vi "Graph of Function and Derivative.vi"() -> ()   [LabVIEW 2020, in "Examples.lvlib"]
doc: "A simple example demonstrating the easiness and usefulness of being able to calculate the derivative of a function automatically, even exchanging which function to differentiate at run-time. This example shows the graph of two different functions and plots the tangent line to the curve at the location of the cursor."
uses:
  Examples.lvlib
  classes/Dual/Dual.lvclass/Dual.ctl
  classes/Dual/Dual to Double.vi
  Automatic Differentiation/Evaluate Function.vi/9b1629ae-3de0-49eb-9b0a-cc9e581fb6c0.vi
  classes/Dual/Add infinitesimal to Double.vi
  classes/Dual/Read Dual Part.vi
  Automatic Differentiation/Evaluate Function.vi/9b1629ae-3de0-49eb-9b0a-cc9e581fb6c0.vi/5957e011-cf56-4527-b6ed-13c3a4ca997b.vi
  classes/Dual/Write a.vi
  Quadratic Function.vi
  Cubic Function.vi
  classes/Dual/Dual.lvclass
  Automatic Differentiation/Automatic Differentiation.lvlib
panel:
  in  "Toggle Function":bool
  in  "Stop":bool
  out "XY Graph":cluster{dbl[], dbl[]}[](graph)
  # "1) Run the VI\n2) Grab and move the cursor and view the graph of the tangent line changing\n3) Toggle f(x) to change the function at run-time\n4) Inspect the block diagram"
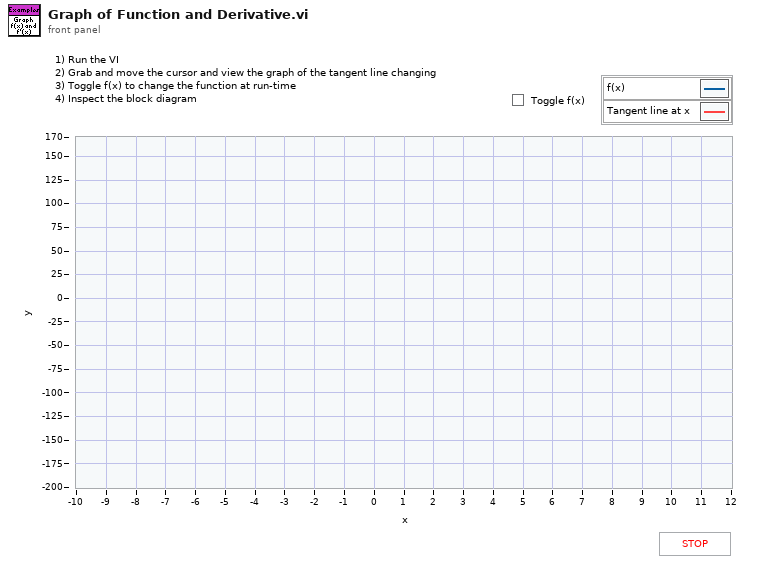
[diagram p1: front panel]
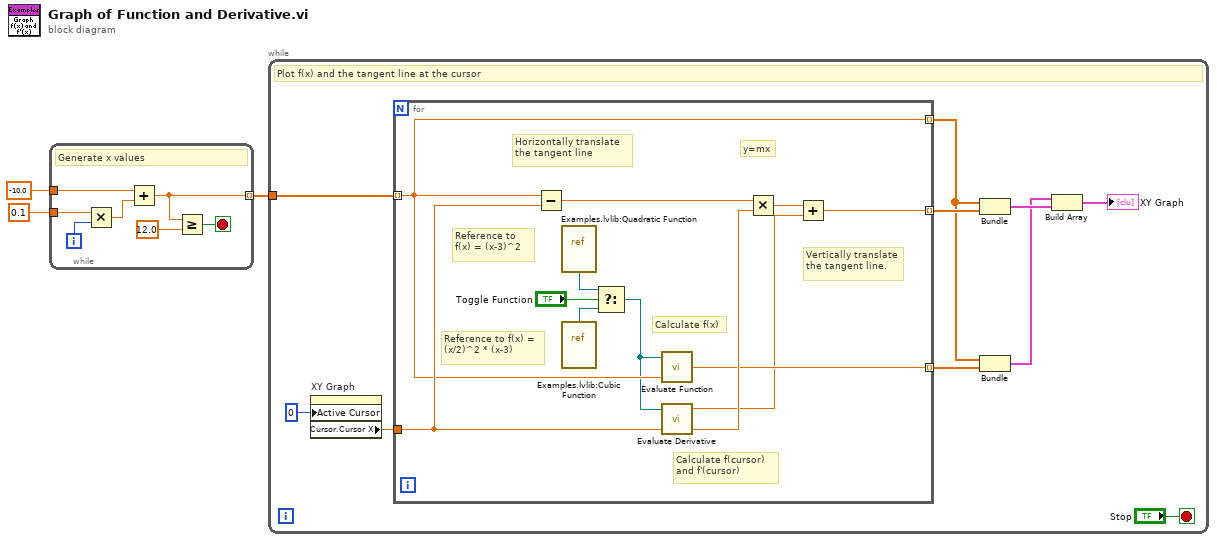
[diagram p0: block diagram]
diagram:
  n1 = while {
    tunnel: -10.0 -> [w7]
    tunnel: 0.1 -> [w9]
    tunnel: [w6] -> w1 mode=indexing
    i -> [w10]
    stop <- w4 stop-if-true
    # "Generate x values"
    n2 = Multiply(x=w9, y=w10) -> (x*y=w8:dbl)
    n3 = Add(x=w7, y=w8) -> (x+y=w6:dbl)
    n4 = Greater Or Equal?(x=w6, y=12.0) -> (x >= y?=w4:bool)
  }
  n5 = while {
    tunnel: w1 -> [w15]
    stop <- "Stop" stop-if-true
    # "Plot f(x) and the tangent line at the cursor"
    n6 = property on="XY Graph" class="XYGraph (strict)"("Active Cursor"=u32 0) -> ("Cursor.Cursor X"=w19:dbl)  [unwired: 2 in, 2 out]
    n7 = for {
      tunnel: w19 -> [w30]
      tunnel: [w28] -> w17 mode=indexing
      tunnel: w15 -> [w27] mode=indexing
      tunnel: [w26] -> w14 mode=indexing
      tunnel: [w27] -> w13 mode=indexing
      # "Reference to f(x) = (x/2)^2 * (x-3)"
      # "y=mx"
      # "Vertically translate the tangent line."
      # "Horizontally translate the tangent line"
      # "Reference to f(x) = (x-3)^2"
      # "Calculate f(x)"
      # "Calculate f(cursor) and f'(cursor)"
      n8 = Subtract(x=w27, y=w30) -> (x-y=w31:dbl)
      n9 = vi-ref "Examples.lvlib:Quadratic Function.vi"() -> (w23:refnum<vi>)
      n10 = vi-ref "Examples.lvlib:Cubic Function.vi"() -> (w22:refnum<vi>)
      n11 = Select(t=w23, s="Toggle Function", f=w22) -> (s? t:f=w21:refnum<vi>)
      n12 = call "Evaluate Function.vi"("x"=w27, "Function Reference"=w21) -> ("f(x)"=w26:dbl)  [unwired: 1 in]
      n13 = call "Evaluate Derivative.vi"("x"=w30, "Function Reference"=w21) -> ("f'(x)"=w32:dbl, "f(x)"=w25:dbl)  [unwired: 2 in]
      n14 = Multiply(x=w31, y=w32) -> (x*y=w29:dbl)
      n15 = Add(x=w29, y=w25) -> (x+y=w28:dbl)
    }
    n16 = Bundle(w13, w17) -> (w16:cluster{dbl[], dbl[]})  [unwired: 1 in]
    n17 = Bundle(w13, w14) -> (w12:cluster{dbl[], dbl[]})  [unwired: 1 in]
    n18 = Build Array(w12, w16) -> (→"XY Graph":cluster{dbl[], dbl[]}[])
  }
